vi "Logger-Set Offset.vi"(7 "Offset":dbl, 11 "error in (no error)":errorcluster) -> (15 "error out":errorcluster)   [LabVIEW 2020]
uses:
  Typedefs/Logger-Queue Data.ctl
  Typedefs/Logger-Action.ctl
  Typedefs/Logger-Level.ctl
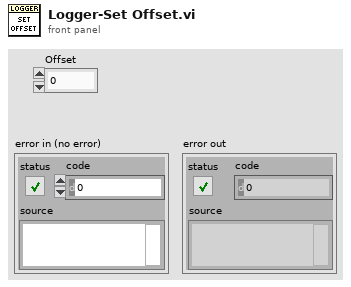
[diagram p1: front panel]
types:
  T1 = typedef "Logger-Action.ctl" = enum16{"None", "Init", "Add", "Show", "Offset", "Quit"}
  T2 = typedef "Logger-Queue Data.ctl" = cluster{"Action":T1, "Level":T3, "Time":dbl, "Message":string}
  T3 = typedef "Logger-Level.ctl" = enum16{"Debug", "TCP", "Info", "Warning", "Error", "Critical"}
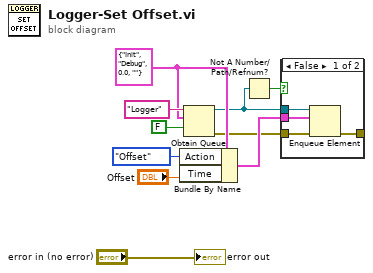
[diagram p0: block diagram]
diagram:
  w8 = T2 {"Action"=enum."Init", "Level"=enum."Debug", "Time"=0.0, "Message"=""} ("Trace Data")
  n1 = Bundle By Name(cluster=w8, "Action"=Logger-Action."Offset", "Time"="Offset") -> (w5:T2)
  n2 = Obtain Queue(name (unnamed)="Logger", element data type=w8, create if not found? (T)=FALSE) -> (queue out=w3:refnum<queue>, error out=w4:errorcluster)  [unwired: 2 in, 1 out]
  n3 = Not A Number/Path/Refnum?(number/path/refnum=w3) -> (NaN/Path/Refnum?=w2:bool)
  n4 = case shown="False" w2 {
    tunnel: w5 -> [w14 _]
    tunnel: w4 -> [w13 _]
    tunnel: w3 -> [w12 _]
    tunnel: [w11 _] -> _
    frame False {
      n5 = Enqueue Element(queue=w12, element=w14, error in (no error)=w13) -> (error out=w11:errorcluster)  [unwired: 1 in, 2 out]
    }
    frame True {
    }
  }
  "error out" <- "error in (no error)"
